vi "Vision Processing.vi"(4 "error in (no error)":errorcluster, 7 "Image Size":T1=enum."320x240") -> ()   [LabVIEW 2014]
doc: "This VI runs in parallel to other tasks. It gets images from the camera, processes them for color or shape and use that information to affect robot behavior."
uses:
  <vilib>/Rock Robotics/WPI/Camera/WPI_CameraImageSize.ctl
  <vilib>/Rock Robotics/WPI/Camera/WPI_CameraWhite Balance Values.ctl
  <vilib>/Rock Robotics/WPI/Camera/WPI_CameraExposure Values.ctl
  <vilib>/Rock Robotics/WPI/Camera/WPI_CameraFrameRate.ctl
  Robot Global Data.vi
panel:
  in  "Image Size 2":T1=enum."320x240"
  in  "error in (no error) 2":errorcluster
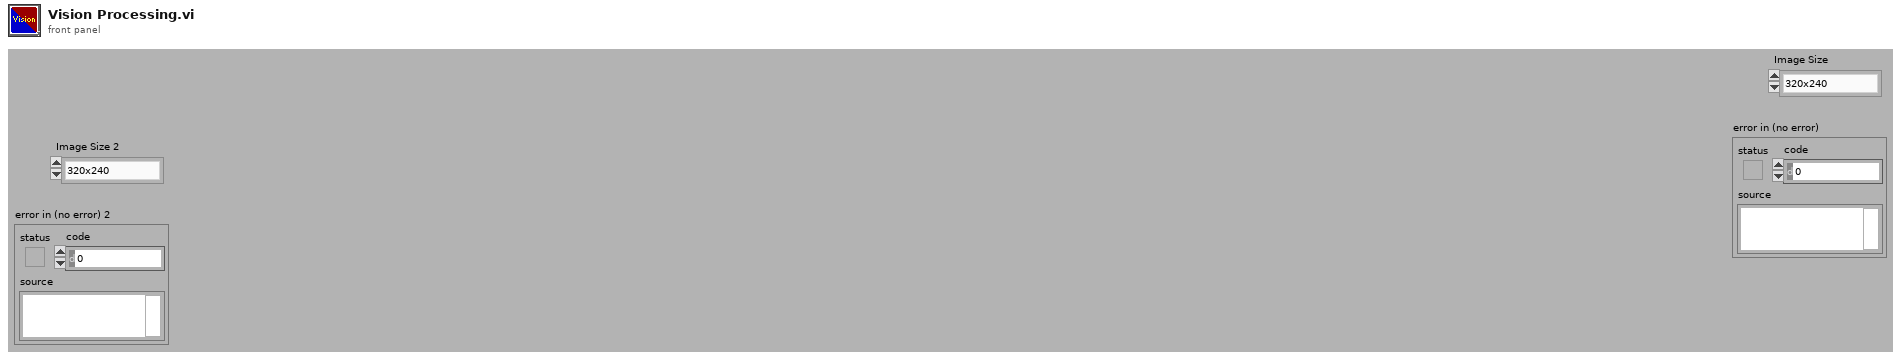
[diagram p1: front panel]
types:
  T1 = typedef "WPI_CameraImageSize.ctl" = enum16{"640x480", "320x240", "160x120", "Custom"}
  T2 = typedef "WPI_CameraFrameRate.ctl" = u32
  T3 = typedef "WPI_CameraExposure Values.ctl" = enum16{"Auto", "Flicker-free 50 Hz", "Flicker-free 60 Hz", "Hold current", "Custom"}
  T4 = typedef "WPI_CameraWhite Balance Values.ctl" = enum16{"Auto", "Fixed indoor", "Fixed outdoor 1", "Fixed outdoor 2", "Fixed fluorescent 1", "Fixed fluorescent 2", "Hold current", "Custom"}
  T5 = typedef "Image Type" = u32
  T6 = typedef "WPI_CameraDevRef.ctl" = cluster{"Camera Address":string, "CameraStatus":errorcluster}
  T7 = typedef "IMAQ Image.ctl" = refnum<image>
  T8 = cluster{"Global Rectangle":cluster{"x1Left":i32, "y1Top":i32, "x2Right":i32, "y2Bottom":i32}, "Centroid":cluster{"x":sgl, "y":sgl}, "Object Size":u32, "Score":dbl}[]
  T9 = typedef "IMAQ GM Match Report.ctl" = cluster{"Position":cluster{"x":sgl, "y":sgl}, "Angle":sgl, "Scale":sgl, "Score":sgl, "Bounding Box":cluster{"x":sgl, "y":sgl}[], "Contrast Reversed":bool, "Occlusion %":sgl, "Template Target Curve Score":sgl, "Target Template Curve Score":sgl, "Correlation Score":sgl}
  T10 = cluster{"Shape Report (calibrated)[0]":cluster{"Global Rectangle":cluster{"x1Left":i32, "y1Top":i32, "x2Right":i32, "y2Bottom":i32}, "Centroid":cluster{"x":sgl, "y":sgl}, "Object Size":u32, "Score":dbl}, "Shape Report (calibrated)[1]":cluster{"Global Rectangle":cluster{"x1Left":i32, "y1Top":i32, "x2Right":i32, "y2Bottom":i32}, "Centroid":cluster{"x":sgl, "y":sgl}, "Object Size":u32, "Score":dbl}, "Shape Report (calibrated)[2]":cluster{"Global Rectangle":cluster{"x1Left":i32, "y1Top":i32, "x2Right":i32, "y2Bottom":i32}, "Centroid":cluster{"x":sgl, "y":sgl}, "Object Size":u32, "Score":dbl}, "Shape Report (calibrated)[3]":cluster{"Global Rectangle":cluster{"x1Left":i32, "y1Top":i32, "x2Right":i32, "y2Bottom":i32}, "Centroid":cluster{"x":sgl, "y":sgl}, "Object Size":u32, "Score":dbl}, "Shape Report (calibrated)[4]":cluster{"Global Rectangle":cluster{"x1Left":i32, "y1Top":i32, "x2Right":i32, "y2Bottom":i32}, "Centroid":cluster{"x":sgl, "y":sgl}, "Object Size":u32, "Score":dbl}, "Shape Report (calibrated)[5]":cluster{"Global Rectangle":cluster{"x1Left":i32, "y1Top":i32, "x2Right":i32, "y2Bottom":i32}, "Centroid":cluster{"x":sgl, "y":sgl}, "Object Size":u32, "Score":dbl}, "Shape Report (calibrated)[6]":cluster{"Global Rectangle":cluster{"x1Left":i32, "y1Top":i32, "x2Right":i32, "y2Bottom":i32}, "Centroid":cluster{"x":sgl, "y":sgl}, "Object Size":u32, "Score":dbl}, "Shape Report (calibrated)[7]":cluster{"Global Rectangle":cluster{"x1Left":i32, "y1Top":i32, "x2Right":i32, "y2Bottom":i32}, "Centroid":cluster{"x":sgl, "y":sgl}, "Object Size":u32, "Score":dbl}, "Shape Report (calibrated)[8]":cluster{"Global Rectangle":cluster{"x1Left":i32, "y1Top":i32, "x2Right":i32, "y2Bottom":i32}, "Centroid":cluster{"x":sgl, "y":sgl}, "Object Size":u32, "Score":dbl}}
  T11 = cluster{"Global Rectangle":cluster{"x1Left":i32, "y1Top":i32, "x2Right":i32, "y2Bottom":i32}, "Centroid":cluster{"x":sgl, "y":sgl}, "Object Size":u32, "Score":dbl}
  T12 = cluster{"Results (Pixels)[0]":sgl, "Results (Pixels)[1]":sgl, "Results (Pixels)[2]":sgl, "Results (Pixels)[3]":sgl, "Results (Pixels)[4]":sgl, "Results (Pixels)[5]":sgl, "Results (Pixels)[6]":sgl, "Results (Pixels)[7]":sgl, "Results (Pixels)[8]":sgl}
  T13 = cluster{"x1Left":i32, "y1Top":i32, "x2Right":i32, "y2Bottom":i32}
  T14 = cluster{"Results (Calibrated)[0]":sgl, "Results (Calibrated)[1]":sgl, "Results (Calibrated)[2]":sgl, "Results (Calibrated)[3]":sgl, "Results (Calibrated)[4]":sgl, "Results (Calibrated)[5]":sgl, "Results (Calibrated)[6]":sgl, "Results (Calibrated)[7]":sgl, "Results (Calibrated)[8]":sgl}
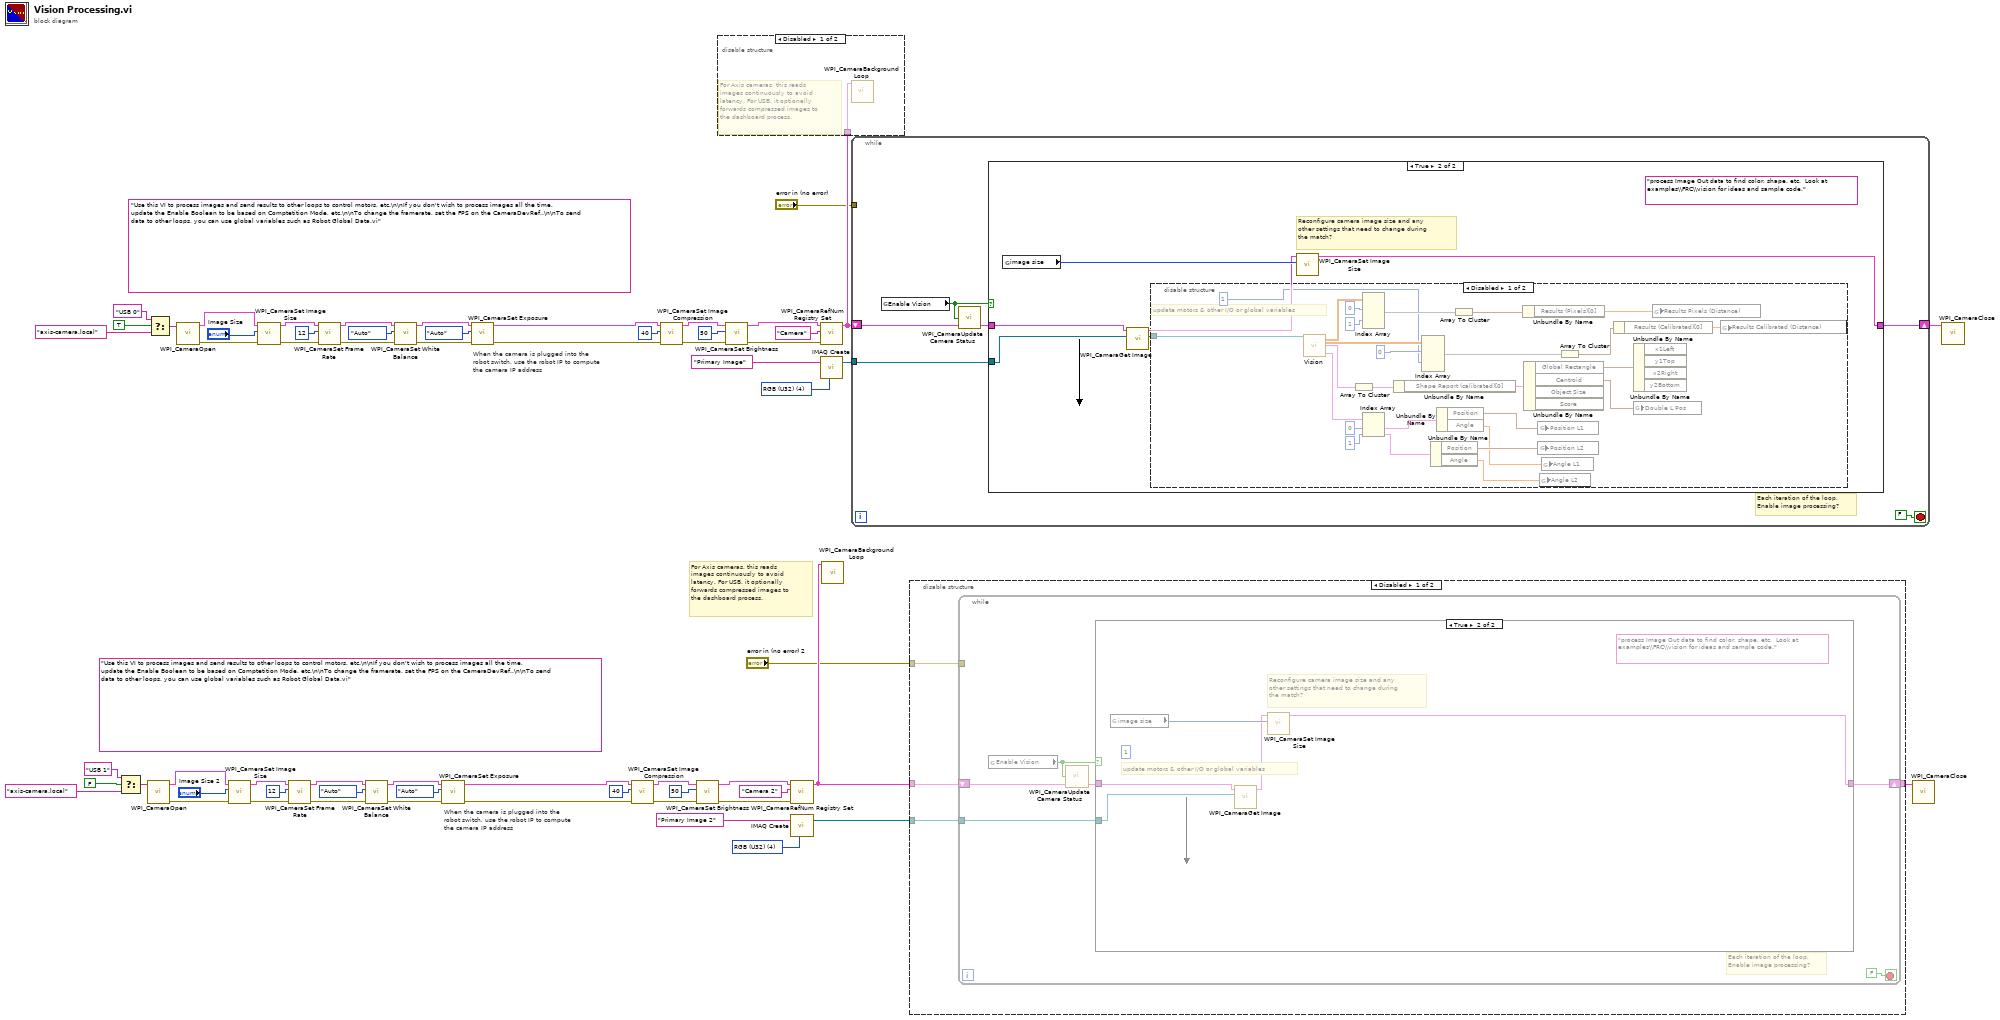
[diagram p0: block diagram]
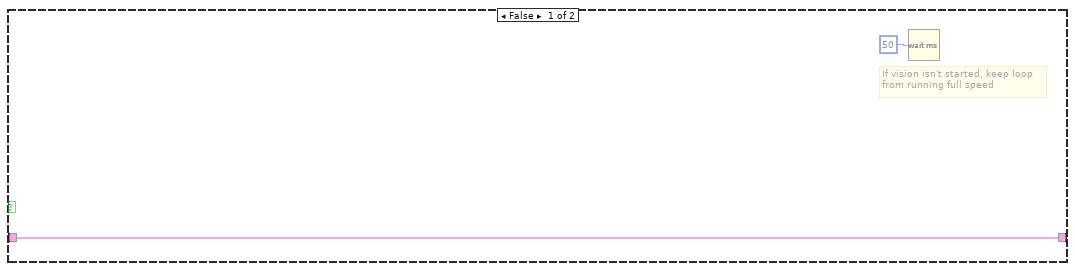
[diagram p3: hidden frame]
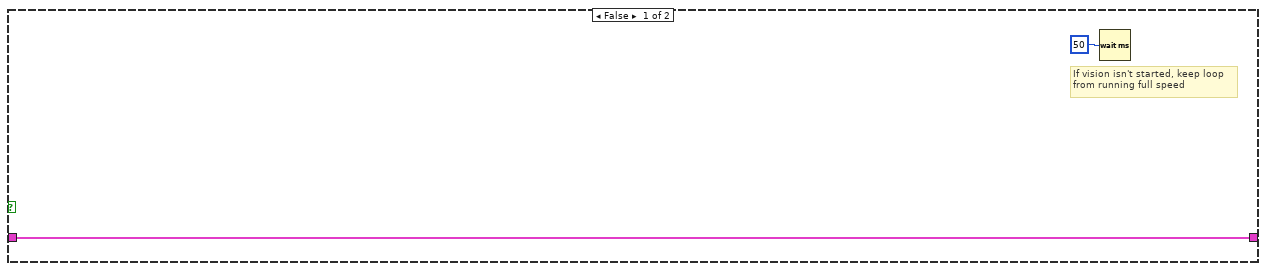
[diagram p5: hidden frame]
diagram:
  (unwired) "Use this VI to process images and send results to other loops to control motors, etc.\n\nIf you don't wish to process images all the time, update the Enable Boolean to be based on Comptetition Mode, etc.\n\nTo change the framerate, set the FPS on the CameraDevRef..\n\nTo send data to other loops, you can use global variables such as Robot Global Data.vi"
  w31 = T5 4 items=["Grayscale (U8)", "Grayscale (I16)", "Grayscale (SGL)", "Complex (CSG)", "RGB (U32)", "HSL (U32)", "RGB (U64)"] ("Image Type")
  (unwired) "Use this VI to process images and send results to other loops to control motors, etc.\n\nIf you don't wish to process images all the time, update the Enable Boolean to be based on Comptetition Mode, etc.\n\nTo change the framerate, set the FPS on the CameraDevRef..\n\nTo send data to other loops, you can use global variables such as Robot Global Data.vi"
  w62 = T5 4 items=["Grayscale (U8)", "Grayscale (I16)", "Grayscale (SGL)", "Complex (CSG)", "RGB (U32)", "HSL (U32)", "RGB (U64)"] ("Image Type")
  # "When the camera is plugged into the\nrobot switch, use the robot IP to compute\nthe camera IP address"
  # "For Axis cameras, this reads\nimages continuously to avoid\nlatency. For USB, it optionally\nforwards compressed images to\nthe dashboard process."
  # "When the camera is plugged into the\nrobot switch, use the robot IP to compute\nthe camera IP address"
  n1 = Select(t="USB 1" ("format string"), s=FALSE ("dot notation? (F)"), f="axis-camera.local" ("format string")) -> (s? t:f=w2:string)
  n2 = call <vilib>:"WPI_CameraOpen.vi"("Camera Address"=w2) -> ("error out"=w19:errorcluster, "CameraDevRef"=w20:T6)  [unwired: 1 in, 8 out]
  n3 = Select(t="USB 0" ("format string"), s=TRUE ("dot notation? (F)"), f="axis-camera.local" ("format string")) -> (s? t:f=w33:string)
  n4 = call <vilib>:"WPI_CameraOpen.vi"("Camera Address"=w33) -> ("error out"=w50:errorcluster, "CameraDevRef"=w51:T6)  [unwired: 1 in, 8 out]
  n5 = call <vilib>:"WPI_CameraSet Image Size.vi"("error in (no error)"=w19, "Image Size"="Image Size 2", "CameraDevRef"=w20) -> ("error out"=w18:errorcluster, "CameraDevRef Out"=w21:T6)  [unwired: 1 in, 6 out]
  n6 = call <vilib>:"WPI_CameraSet Image Size.vi"("error in (no error)"=w50, "Image Size"="Image Size", "CameraDevRef"=w51) -> ("error out"=w49:errorcluster, "CameraDevRef Out"=w52:T6)  [unwired: 1 in, 6 out]
  n7 = call <vilib>:"WPI_CameraSet Frame Rate.vi"("error in (no error)"=w18, "Frame Rate (fps)"=T2 12, "CameraDevRef"=w21) -> ("error out"=w17:errorcluster, "CameraDevRef Out"=w23:T6)  [unwired: 7 out]
  n8 = call <vilib>:"WPI_CameraSet Frame Rate.vi"("error in (no error)"=w49, "Frame Rate (fps)"=T2 12, "CameraDevRef"=w52) -> ("error out"=w48:errorcluster, "CameraDevRef Out"=w54:T6)  [unwired: 7 out]
  n9 = call <vilib>:"WPI_CameraSet White Balance.vi"("error in (no error)"=w17, "White Balance"=WPI_CameraWhite_Balance_Values."Auto", "CameraDevRef"=w23) -> ("error out"=w16:errorcluster, "CameraDevRef Out"=w22:T6)  [unwired: 1 in, 6 out]
  n10 = call <vilib>:"WPI_CameraSet White Balance.vi"("error in (no error)"=w48, "White Balance"=WPI_CameraWhite_Balance_Values."Auto", "CameraDevRef"=w54) -> ("error out"=w47:errorcluster, "CameraDevRef Out"=w53:T6)  [unwired: 1 in, 6 out]
  n11 = call <vilib>:"WPI_CameraSet Exposure.vi"("error in (no error)"=w16, "Exposure"=WPI_CameraExposure_Values."Auto", "CameraDevRef"=w22) -> ("error out"=w15:errorcluster, "CameraDevRef Out"=w25:T6)  [unwired: 1 in, 6 out]
  n12 = call <vilib>:"WPI_CameraSet Exposure.vi"("error in (no error)"=w47, "Exposure"=WPI_CameraExposure_Values."Auto", "CameraDevRef"=w53) -> ("error out"=w46:errorcluster, "CameraDevRef Out"=w56:T6)  [unwired: 1 in, 6 out]
  n13 = call <vilib>:"WPI_CameraSet Image Compression.vi"("error in (no error)"=w15, "Compression"=40, "CameraDevRef"=w25) -> ("error out"=w14:errorcluster, "CameraDevRef Out"=w24:T6)  [unwired: 7 out]
  n14 = call <vilib>:"WPI_CameraSet Image Compression.vi"("error in (no error)"=w46, "Compression"=40, "CameraDevRef"=w56) -> ("error out"=w45:errorcluster, "CameraDevRef Out"=w55:T6)  [unwired: 7 out]
  n15 = call <vilib>:"WPI_CameraSet Brightness.vi"("error in (no error)"=w14, "Brightness"=50, "CameraDevRef"=w24) -> ("error out"=w12:errorcluster, "CameraDevRef Out"=w13:T6)  [unwired: 7 out]
  n16 = call <vilib>:"WPI_CameraSet Brightness.vi"("error in (no error)"=w45, "Brightness"=50, "CameraDevRef"=w55) -> ("error out"=w43:errorcluster, "CameraDevRef Out"=w44:T6)  [unwired: 7 out]
  n17 = call <vilib>:"WPI_CameraRefNum Registry Set.vi"("error in (no error)"=w12, "refnum name"="Camera 2", "CameraDevRef"=w13) -> ("CameraDevRef"=w8:T6)  [unwired: 8 out]
  n18 = call "IMAQ Create"("Image Name"="Primary Image 2", "Image Type"=w31) -> ("New Image"=w29:T7)  [unwired: 2 in, 2 out]
  n19 = call <vilib>:"WPI_CameraRefNum Registry Set.vi"("error in (no error)"=w43, "refnum name"="Camera", "CameraDevRef"=w44) -> ("CameraDevRef"=w39:T6)  [unwired: 8 out]
  n20 = disable-structure shown="Disabled" {
    disable-tunnel: w39 -> [w63 _]
    frame Disabled {
      # "For Axis cameras, this reads\nimages continuously to avoid\nlatency. For USB, it optionally\nforwards compressed images to\nthe dashboard process."
      n21 = call <vilib>:"WPI_CameraBackground Loop.vi"("CameraDevRef"=w63) -> ()  [unwired: 11 in]
    }
    frame Enabled {
    }
  }
  n22 = call "IMAQ Create"("Image Name"="Primary Image", "Image Type"=w62) -> ("New Image"=w60:T7)  [unwired: 2 in, 2 out]
  n23 = call <vilib>:"WPI_CameraBackground Loop.vi"("CameraDevRef"=w8) -> ()  [unwired: 11 in]
  n24 = while {
    shift-right: [w68] -> w37
    shift-left: w39 -> [w66]
    tunnel: w60 -> [w67]
    tunnel: "error in (no error)" -> [_]
    stop <- FALSE stop-if-true
    # "Each iteration of the loop,\nEnable image processing?"
    n25 = global read "Robot Global Data.vi" "Enable Vision"() -> (w64:bool)
    n26 = call <vilib>:"WPI_CameraUpdate Camera Status.vi"("CameraDevRef In"=w66, "Enable Vision"=w64) -> ("CameraDevRef Out"=w65:T6)  [unwired: 3 in]
    n27 = case shown="True" w64 {
      tunnel: w67 -> [_ w76]
      tunnel: [w71 w77] -> w68
      tunnel: w65 -> [w71 w74]
      frame False {
        # "If vision isn't started, keep loop\nfrom running full speed"
        n28 = Wait (ms)(milliseconds to wait=u32 50) -> ()  [unwired: 1 out]
      }
      frame True {
        (unwired) "process Image Out data to find color, shape, etc.  Look at examples\\FRC\\vision for ideas and sample code."
        # "Reconfigure camera image size and any\nother settings that need to change during\nthe match?"
        n29 = global read "Robot Global Data.vi" "image size"() -> (w75:T1)
        n30 = call <vilib>:"WPI_CameraGet Image.vi"("Image"=w76, "CameraDevRef"=w74) -> ("Image Out"=w72:T7, "CameraDevRef Out"=w73:T6)  [unwired: 1 in, 7 out]
        n31 = disable-structure shown="Disabled" {
          disable-tunnel: w72 -> [w104 _]
          frame Disabled {
            # "update motors & other I/O or global variables"
            n32 = call "Vision.vi"("Image In"=w104) -> ("Results (Pixels)"=w98:sgl[][], "Results (Calibrated)"=w92:sgl[][], "Shape Report (calibrated)"=w103:T8, "Calibrated Matches"=w87:T9[])  [unwired: 21 in, 2 out]
            n33 = Array To Cluster(array=w103) -> (cluster=w102:T10)
            n34 = Index Array(array=w98, index (row) #1=0 ("index (row)"), index (row) #2=1 ("index (row)")) -> (element #1=w95:sgl[])  [unwired: 2 in, 1 out]
            n35 = Index Array(array=w87, index #1=0 ("index"), index #2=1 ("index")) -> (element #1=w84:T9, element #2=w83:T9)
            n36 = Unbundle By Name(w102) -> ("Shape Report (calibrated)[0]"=w101:T11)
            n37 = Index Array(array=w92, index (row) #1=0 ("index (row)"), index (row) #2=1 ("index (row)")) -> (element #1=w90:sgl[])  [unwired: 2 in, 1 out]
            n38 = Unbundle By Name(w83) -> ("Position"=w81:cluster{"x":sgl, "y":sgl}, "Angle"=w79:sgl)
            n39 = Unbundle By Name(w84) -> ("Position"=w82:cluster{"x":sgl, "y":sgl}, "Angle"=w80:sgl)
            n40 = Array To Cluster(array=w95) -> (cluster=w94:T12)
            n41 = Unbundle By Name(w94) -> ("Results (Pixels)[0]"=w93:sgl)
            n42 = Unbundle By Name(w101) -> ("Global Rectangle"=w100:T13, "Centroid"=w99:cluster{"x":sgl, "y":sgl})  [unwired: 2 out]
            n43 = global write "Robot Global Data.vi" "Position L1"(w82) -> ()
            n44 = global write "Robot Global Data.vi" "Position L2"(w81) -> ()
            n45 = global write "Robot Global Data.vi" "Angle L2"(w79) -> ()
            n46 = global write "Robot Global Data.vi" "Angle L1"(w80) -> ()
            n47 = Array To Cluster(array=w90) -> (cluster=w89:T14)
            n48 = Unbundle By Name(w89) -> ("Results (Calibrated)[0]"=w88:sgl)
            n49 = Unbundle By Name(w100) -> ()  [unwired: 4 out]
            n50 = global write "Robot Global Data.vi" "Double L Pos"(w99) -> ()
            n51 = global write "Robot Global Data.vi" "Results Pixels (Distance)"(w93) -> ()
            n52 = global write "Robot Global Data.vi" "Results Calibrated (Distance)"(w88) -> ()
          }
          frame Enabled {
          }
        }
        n53 = call <vilib>:"WPI_CameraSet Image Size.vi"("Image Size"=w75, "CameraDevRef"=w73) -> ("CameraDevRef Out"=w77:T6)  [unwired: 2 in, 7 out]
      }
    }
  }
  n54 = disable-structure shown="Disabled" {
    disable-tunnel: w29 -> [w108 _]
    disable-tunnel: w8 -> [w107 _]
    disable-tunnel: [w106 _] -> w6
    disable-tunnel: "error in (no error) 2" -> [w105 _]
    frame Disabled {
      n55 = while {
        shift-right: [w113] -> w106
        shift-left: w107 -> [w111]
        tunnel: w108 -> [w112]
        tunnel: w105 -> [_]
        stop <- FALSE stop-if-true
        # "Each iteration of the loop,\nEnable image processing?"
        n56 = global read "Robot Global Data.vi" "Enable Vision"() -> (w109:bool)
        n57 = call <vilib>:"WPI_CameraUpdate Camera Status.vi"("CameraDevRef In"=w111, "Enable Vision"=w109) -> ("CameraDevRef Out"=w110:T6)  [unwired: 3 in]
        n58 = case shown="True" w109 {
          tunnel: w112 -> [_ w120]
          tunnel: [w116 w121] -> w113
          tunnel: w110 -> [w116 w118]
          frame False {
            # "If vision isn't started, keep loop\nfrom running full speed"
            n59 = Wait (ms)(milliseconds to wait=u32 50) -> ()  [unwired: 1 out]
          }
          frame True {
            (unwired) 1 ("index (row)")
            (unwired) "process Image Out data to find color, shape, etc.  Look at examples\\FRC\\vision for ideas and sample code."
            # "update motors & other I/O or global variables"
            # "Reconfigure camera image size and any\nother settings that need to change during\nthe match?"
            n60 = global read "Robot Global Data.vi" "image size"() -> (w119:T1)
            n61 = call <vilib>:"WPI_CameraGet Image.vi"("Image"=w120, "CameraDevRef"=w118) -> ("CameraDevRef Out"=w117:T6)  [unwired: 1 in, 8 out]
            n62 = call <vilib>:"WPI_CameraSet Image Size.vi"("Image Size"=w119, "CameraDevRef"=w117) -> ("CameraDevRef Out"=w121:T6)  [unwired: 2 in, 7 out]
          }
        }
      }
    }
    frame Enabled {
    }
  }
  n63 = call <vilib>:"WPI_CameraClose.vi"("CameraDevRef"=w6) -> ()  [unwired: 1 in, 10 out]
  n64 = call <vilib>:"WPI_CameraClose.vi"("CameraDevRef"=w37) -> ()  [unwired: 1 in, 10 out]
